vi "voltagesensor-1.vi"() -> ()   [LabVIEW 2022 SP3]
uses:
  <vilib>/DAQmx/read.llb/DAQmx Read (Analog 1D DBL NChan 1Samp).vi
  <vilib>/DAQmx/write.llb/DAQmx Write (Digital Bool 1Line 1Point).vi
  <vilib>/DAQmx/create/channels.llb/DAQmx Create Channel (AI-Voltage-Basic).vi
  <vilib>/DAQmx/create/channels.llb/DAQmx Create Channel (DO-Digital Output).vi
  <vilib>/DAQmx/miscellaneous.llb/DAQmx Fill In Error Info.vi
  <vilib>/httpClient/PUTBuffer.vi
  <vilib>/httpClient/LabVIEWHTTPClient.lvlib
panel:
  out "fan and motor":bool
  in  "stop (F)":bool
  out "Square":dynamicdata(graph)
  in  "Frequency":dbl=50.0
  in  "Offset":dbl=2.5
  in  "Amplitude":dbl=2.5
  in  "DAQmx Physical Channel 4":tag
  out "Boolean 2":bool
  out "Boolean":bool
  out "String 2":string
  out "String":string
  out "HUMIDITY":dbl(knob) scale=0.0..60.0
  out "TEMPARATURE":dbl(slide) scale=0.0..100.0
  out "Temparature":dbl(graph)
  in  "Cluster":T1
  out "Humadity":dbl(graph)
  in  "DAQmx Physical Channel 2":tag
  out "Waveform Chart":dbl(graph)
  in  "stop":bool
  in  "DAQmx Physical Channel":tag
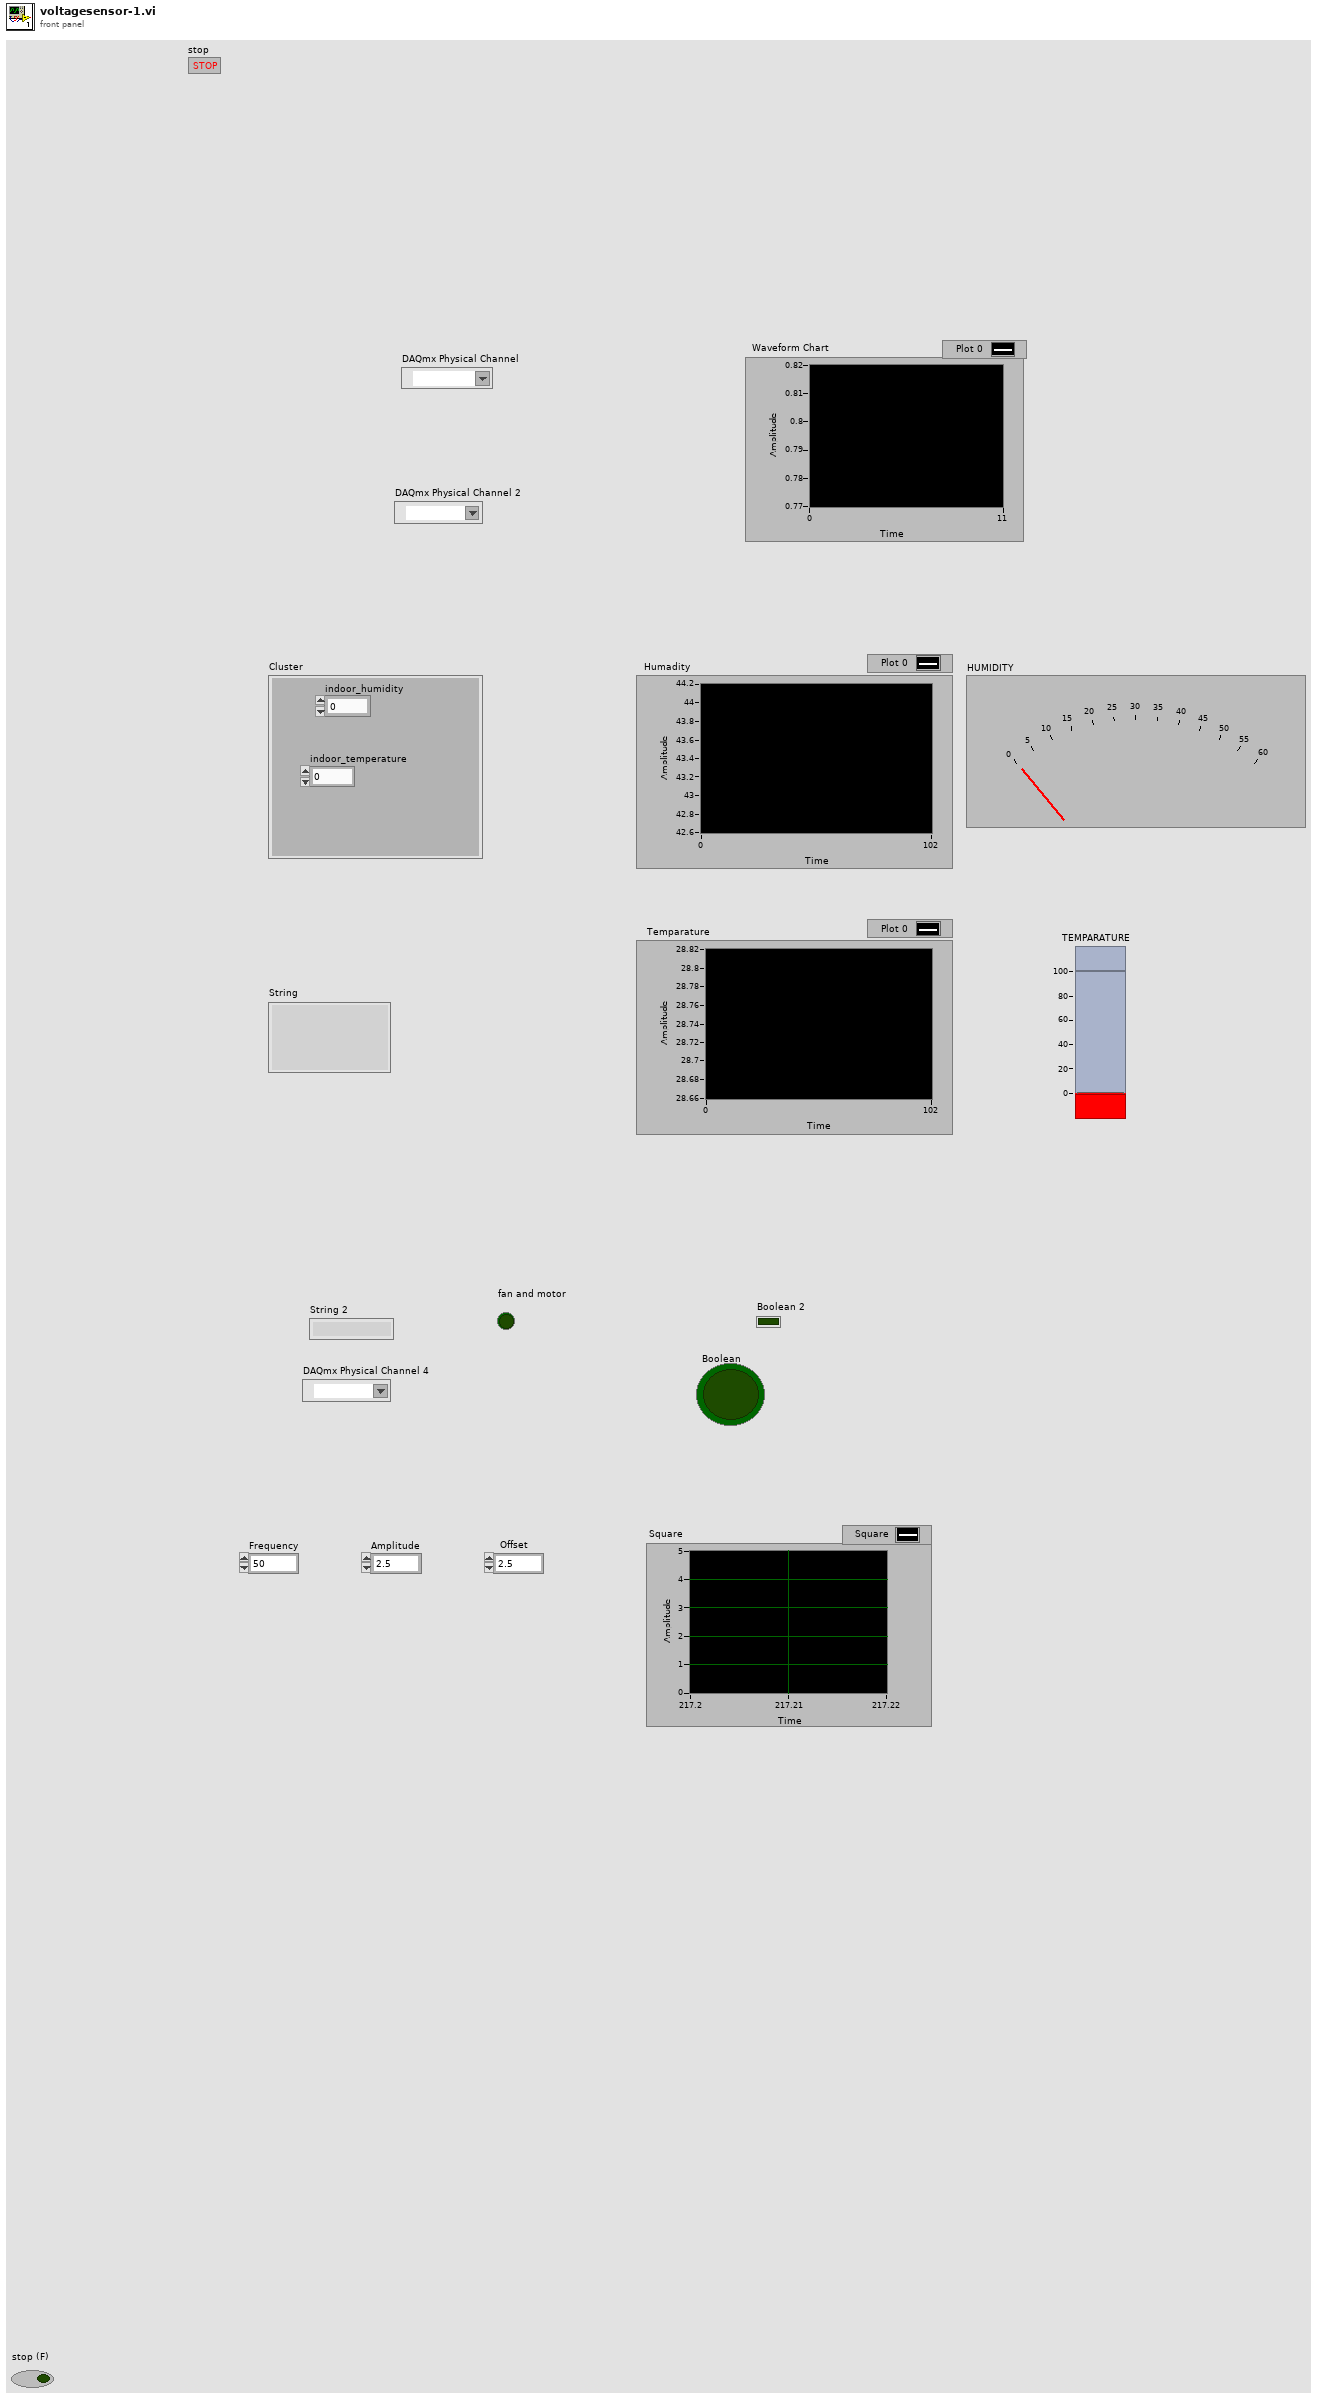
[diagram p1: front panel]
types:
  T1 = cluster{"indoor_humidity":dbl, "indoor_temperature":dbl}
  T2 = typedef "LabVIEWHTTPClient.lvlib/ClientHandle.ctl" = refnum<k1>
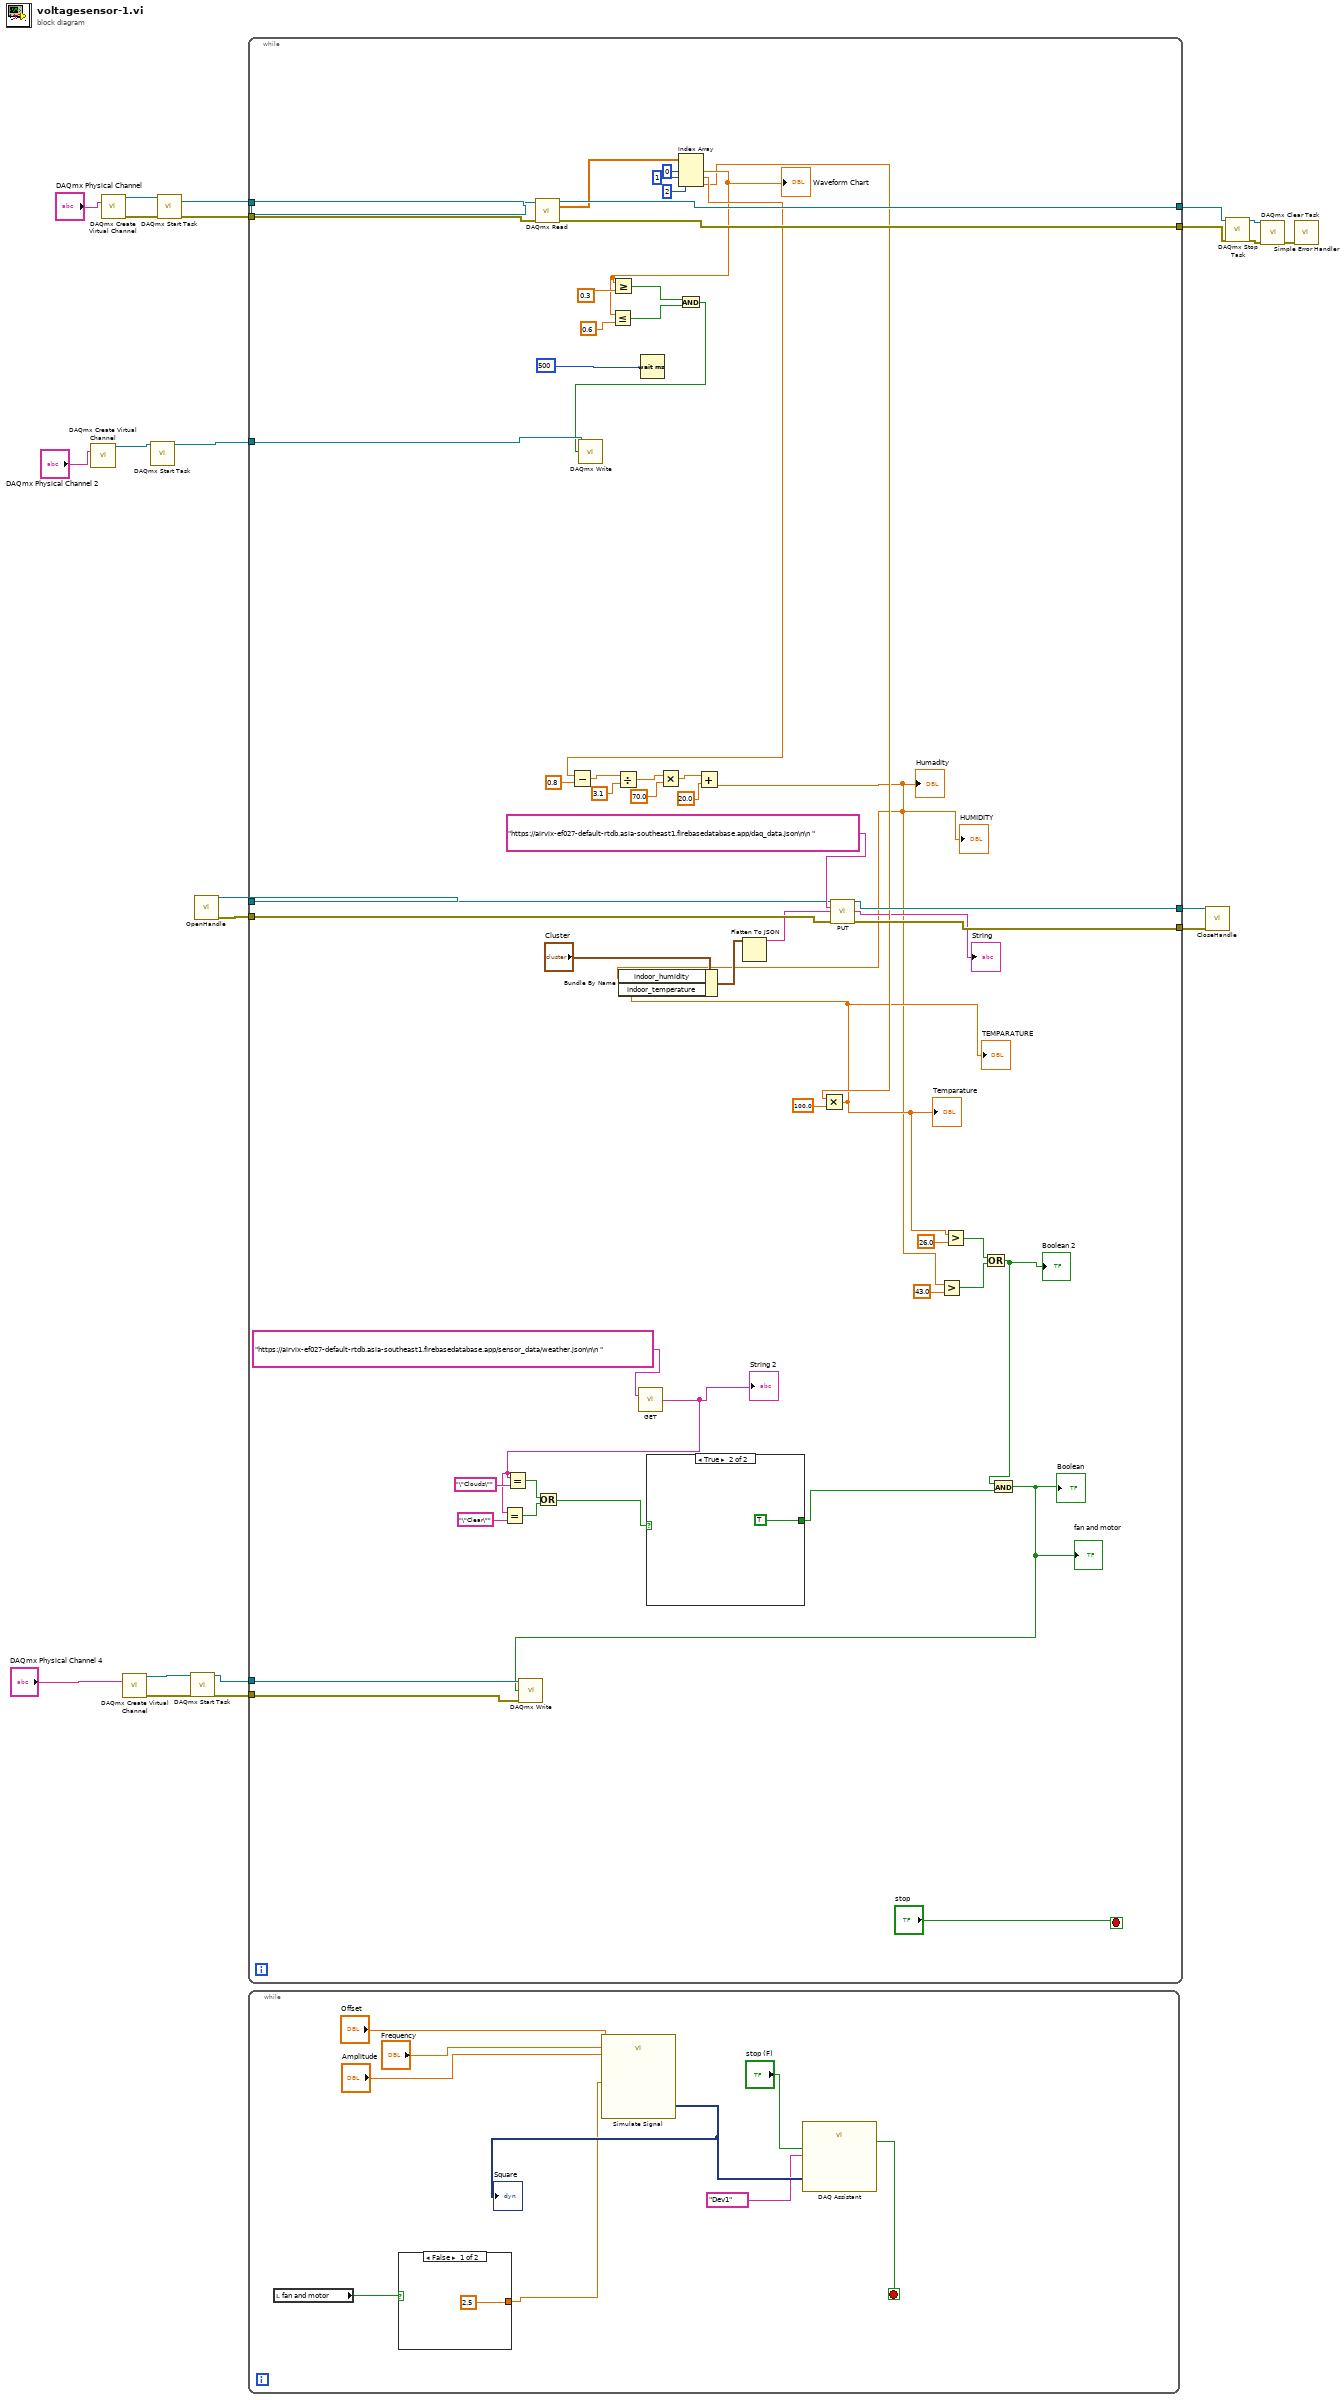
[diagram p0: block diagram]
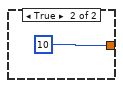
[diagram p2: hidden frame]
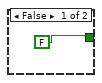
[diagram p3: hidden frame]
diagram:
  n1 = call-poly <vilib>:"DAQmx Create Virtual Channel.vi"("lines"="DAQmx Physical Channel 2") -> ("task out"=w11:refnum<k21>)  [unwired: 13 in, 1 out]
  n2 = call-poly <vilib>:"DAQmx Create Virtual Channel.vi"("physical channels"="DAQmx Physical Channel") -> ("task out"=w20:refnum<k21>, "error out"=w21:errorcluster)  [unwired: 13 in]
  n3 = call-poly <vilib>:"DAQmx Create Virtual Channel.vi"("lines"="DAQmx Physical Channel 4") -> ("task out"=w4:refnum<k21>, "error out"=w2:errorcluster)  [unwired: 13 in]
  n4 = call <vilib>:"DAQmx Start Task.vi"("task/channels in"=w11) -> ("task out"=w10:refnum<k21>)  [unwired: 13 in, 1 out]
  n5 = call <vilib>:"DAQmx Start Task.vi"("task/channels in"=w20, "error in"=w21) -> ("task out"=w13:refnum<k21>, "error out"=w19:errorcluster)  [unwired: 12 in]
  n6 = call <vilib>:"DAQmx Start Task.vi"("task/channels in"=w4, "error in"=w2) -> ("task out"=w3:refnum<k21>, "error out"=w1:errorcluster)  [unwired: 12 in]
  n7 = call <vilib>:"OpenHandle.vi"() -> ("client handle out"=w9:T2, "error out"=w7:errorcluster)  [unwired: 14 in]
  n8 = while {
    tunnel: w13 -> [w76]
    tunnel: w19 -> [w75]
    tunnel: [w73] -> w16
    tunnel: [w74] -> w15
    tunnel: w10 -> [w68]
    tunnel: w9 -> [w59]
    tunnel: [w58] -> w8
    tunnel: w7 -> [w57]
    tunnel: [w56] -> w6
    tunnel: w3 -> [w25]
    tunnel: w1 -> [w24]
    stop <- "stop" stop-if-true
    n9 = call-poly <vilib>:"DAQmx Read.vi"("task/channels in"=w76, "error in"=w75) -> ("task out"=w73:refnum<k21>, "data"=w54:dbl[], "error out"=w74:errorcluster)  [unwired: 11 in]
    n10 = call <vilib>:"GET.vi"("url"="https://airvix-ef027-default-rtdb.asia-southeast1.firebasedatabase.app/sensor_data/weather.json\n\n ") -> ("body"=w35:string)  [unwired: 11 in, 3 out]
    "String 2" <- w35
    n11 = Equal?(x=w35, y="\"Clear\"") -> (x = y?=w37:bool)
    n12 = Equal?(x=w35, y="\"Clouds\"") -> (x = y?=w36:bool)
    n13 = Or(x=w36, y=w37) -> (x .or. y?=w26:bool)
    n14 = Wait (ms)(milliseconds to wait=500) -> ()  [unwired: 1 out]
    n15 = case shown="True" w26 {
      tunnel: [FALSE TRUE] -> w27
      frame False {
      }
      frame True {
      }
    }
    n16 = Index Array "Index Array"(array=w54, index #1=0 ("index"), index #2=1 ("index"), index #3=2 ("index")) -> (element #1=w47:dbl, element #2=w48:dbl, element #3=w42:dbl)
    "Waveform Chart" <- w47
    n17 = Subtract(x=w48, y=0.8) -> (x-y=w66:dbl)
    n18 = Less Or Equal?(x=w47, y=0.6) -> (x <= y?=w50:bool)
    n19 = Greater Or Equal?(x=w47, y=0.3) -> (x >= y?=w51:bool)
    n20 = Divide(x=w66, y=3.1) -> (x/y=w64:dbl)
    n21 = Multiply(x=w64, y=70.0) -> (x*y=w62:dbl)
    n22 = And(x=w51, y=w50) -> (x .and. y?=w49:bool)
    n23 = call-poly <vilib>:"DAQmx Write.vi"("task/channels in"=w68, "data"=w49) -> ()  [unwired: 11 in, 3 out]
    n24 = Add(x=w62, y=20.0) -> (x+y=w31:dbl)
    "Humadity" <- w31
    "HUMIDITY" <- w31
    n25 = Multiply(x=w42, y=100.0) -> (x*y=w32:dbl)
    "Temparature" <- w32
    "TEMPARATURE" <- w32
    n26 = Bundle By Name(cluster="Cluster", "indoor_humidity"=w31, "indoor_temperature"=w32) -> (w46:T1)
    n27 = Flatten To JSON(anything=w46) -> (JSON string=w55:string)  [unwired: 2 in, 1 out]
    n28 = call-poly <vilib>:"PUT.vi"("client handle"=w59, "url"="https://airvix-ef027-default-rtdb.asia-southeast1.firebasedatabase.app/daq_data.json\n\n ", "buffer"=w55, "error in (no error)"=w57) -> ("client handle out"=w58:T2, "body"=→"String":string, "error out"=w56:errorcluster)  [unwired: 8 in, 1 out]
    n29 = Greater?(x=w31, y=43.0) -> (0:w29:bool)
    n30 = Greater?(x=w32, y=26.0) -> (0:w30:bool)
    n31 = Or(x=w30, y=w29) -> (x .or. y?=w28:bool)
    "Boolean 2" <- w28
    n32 = And(x=w28, y=w27) -> (x .and. y?=w23:bool)
    "Boolean" <- w23
    "fan and motor" <- w23
    n33 = call-poly <vilib>:"DAQmx Write.vi"("task/channels in"=w25, "data"=w23, "error in"=w24) -> ()  [unwired: 10 in, 3 out]
  }
  n34 = while {
    stop <- w86 stop-if-true
    n35 = local read "fan and motor"() -> (w80:bool)
    n36 = case shown="False" w80 {
      tunnel: [2.5 10] -> w79
      frame False {
      }
      frame True {
      }
    }
    n37 = call "Simulate Signal"("Offset"="Offset", "Duty Cycle (%)"=w79, "Frequency"="Frequency", "Amplitude"="Amplitude") -> ("Square"=w82:dynamicdata)  [unwired: 10 in, 1 out]
    "Square" <- w82
    n38 = call "DAQ Assistant"("data"=w82, "stop (F)"="stop (F)", "device name"=tag "Dev1") -> ("stopped"=w86:bool)  [unwired: 14 in, 2 out]
  }
  n39 = call <vilib>:"CloseHandle.vi"("client handle"=w8, "error in (no error)"=w6) -> ()  [unwired: 13 in, 1 out]
  n40 = call <vilib>:"DAQmx Stop Task.vi"("task/channels in"=w16, "error in"=w15) -> ("task out"=w18:refnum<k21>, "error out"=w17:errorcluster)  [unwired: 12 in]
  n41 = call <vilib>:"DAQmx Clear Task.vi"("task in"=w18, "error in"=w17) -> ("error out"=w14:errorcluster)  [unwired: 13 in]
  n42 = call <vilib>:"Simple Error Handler.vi"("error in (no error)"=w14) -> ()  [unwired: 4 in, 5 out]
